vi "Get Error (Owner).vi"(8 "error in (no error)":errorcluster, 10 "owner":string, 11 "error list <scope>":variant) -> (0 "error out":errorcluster, 1 "found?":bool, 2 "error list <owner>":variant, 3 "error list <scope> dup":variant)   [LabVIEW 2017]
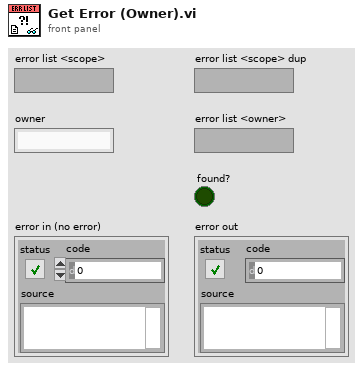
[diagram p1: front panel]
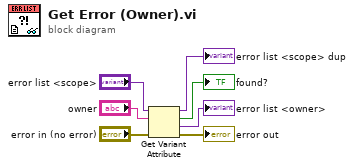
[diagram p0: block diagram]
diagram:
  n1 = Get Variant Attribute(Variant="error list <scope>", name="owner", error in="error in (no error)") -> (duplicate Variant=→"error list <scope> dup":variant, found=→"found?":bool, value=→"error list <owner>":variant, error out=→"error out":errorcluster)  [unwired: 1 in]
